vi "StringArray_Build Time List.vi"(4 "dt":dbl=1.0, 5 "Size":i32) -> (1 "Time Array":string[](array[string]))   [LabVIEW 2020, in "WavBuf.lvclass"]
uses:
  WavBuf/WavBuf.lvclass
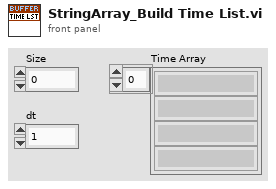
[diagram p1: front panel]
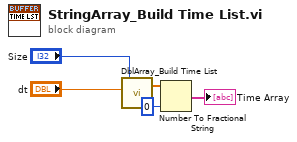
[diagram p0: block diagram]
diagram:
  n1 = call "DblArray_Build Time List.vi"("dt"="dt", "Size"="Size") -> ("Time Array"=w1:dbl[])  [unwired: 3 in]
  n2 = Number To Fractional String(number=w1, precision (6)=i16 0) -> (F-format string=→"Time Array":string[])  [unwired: 2 in]
